vi "GetProperties.vi"(8 "error in":errorcluster, 11 "WaveformChart in":refnum<class "XYGraph.lvclass">) -> (0 "error out":errorcluster, 3 "WaveformChart out":refnum<class "XYGraph.lvclass">)   [LabVIEW 2014, in "XYGraph.lvclass"]
uses:
  XYGraph.lvclass
  XYGraph.lvclass/XYGraph.ctl
  WaveformGraph/WaveformGraph.lvclass
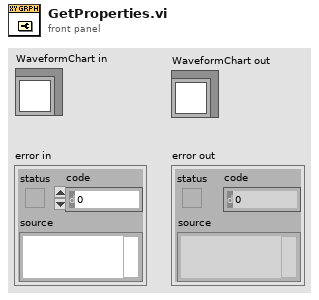
[diagram p1: front panel]
types:
  T1 = enum16{"None", "Nyquist", "Nichols", "S Plane", "Z Plane"}
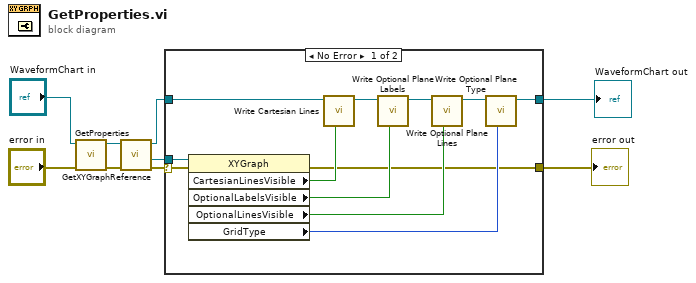
[diagram p0: block diagram]
diagram:
  n1 = call-parent "GetProperties.vi"("error in"="error in", "WaveformChart in"="WaveformChart in") -> ("error out"=w6:errorcluster, "WaveformChart out"=w7:refnum<class "XYGraph.lvclass">)  [unwired: 8 in]
  n2 = call "GetXYGraphReference.vi"("error in"=w6, "XYGraph in"=w7) -> ("error out"=w5:errorcluster, "XYGraph reference"=w4:refnum<vi>, "XYGraph out"=w3:refnum<class "XYGraph.lvclass">)  [unwired: 7 in]
  n3 = case shown="No Error" w5 {
    selector: w5 -> [w20 w22]
    tunnel: w4 -> [w21 _]
    tunnel: w3 -> [w19 w23]
    tunnel: [w11 w23] -> w1
    tunnel: [w10 w22] -> w2
    frame No Error {
      n4 = property class="XYGraph"(reference=w21, error in=w20) -> (error out=w10:errorcluster, "CartesianLinesVisible"=w15:bool, "OptionalLabelsVisible"=w14:bool, "OptionalLinesVisible"=w13:bool, "GridType"=w12:T1)  [unwired: 1 out]
      n5 = call "Write Cartesian Lines .vi"("Cartesian Lines"=w15, "XYGraph in"=w19) -> ("XYGraph out"=w18:refnum<class "XYGraph.lvclass">)  [unwired: 7 in]
      n6 = call "Write Optional Plane Labels.vi"("Optional Plane Labels"=w14, "XYGraph in"=w18) -> ("XYGraph out"=w17:refnum<class "XYGraph.lvclass">)  [unwired: 7 in]
      n7 = call "Write Optional Plane Lines.vi"("Optional Plane Lines"=w13, "XYGraph in"=w17) -> ("XYGraph out"=w16:refnum<class "XYGraph.lvclass">)  [unwired: 7 in]
      n8 = call "Write Optional Plane Type.vi"("Optional Plane Type"=w12, "XYGraph in"=w16) -> ("XYGraph out"=w11:refnum<class "XYGraph.lvclass">)  [unwired: 7 in]
    }
    frame Error {
    }
  }
  "error out" <- w2
  "WaveformChart out" <- w1
